vi "AlliGator Extrapolate Multiple Plots.vi"(8 "error in (no error)":errorcluster, 10 "Selected Plots":i32[](array[numeric]), 11 "Selected Plot Info":T1) -> (0 "error out":errorcluster, 1 "Extrapolated Decay Message":string, 3 "Last Extrapolated Decay":cluster{"t Array":dbl[], "IRF Array":dbl[]}, 4 "Single Plot?":bool)   [LabVIEW 2021, in "AlliGator Decay Processing.lvlib"]
doc: "Extrapolated the selected plots."
uses:
  AlliGator Decay Processing.lvlib
  Graphs/XY Graph/XY Graph Selected Plot Info.ctl
  Graphs/XY Graph/XY Graph Refnum.ctl
  <vilib>/Utility/miscctls.llb/LVPoint32TypeDef.ctl
  Strings/Strings.lvlib
  Decay Preprocessing/AlliGator Decay Preprocessing.lvlib
  Graphs/XY Graph/XY Graph Add-Ons.lvlib
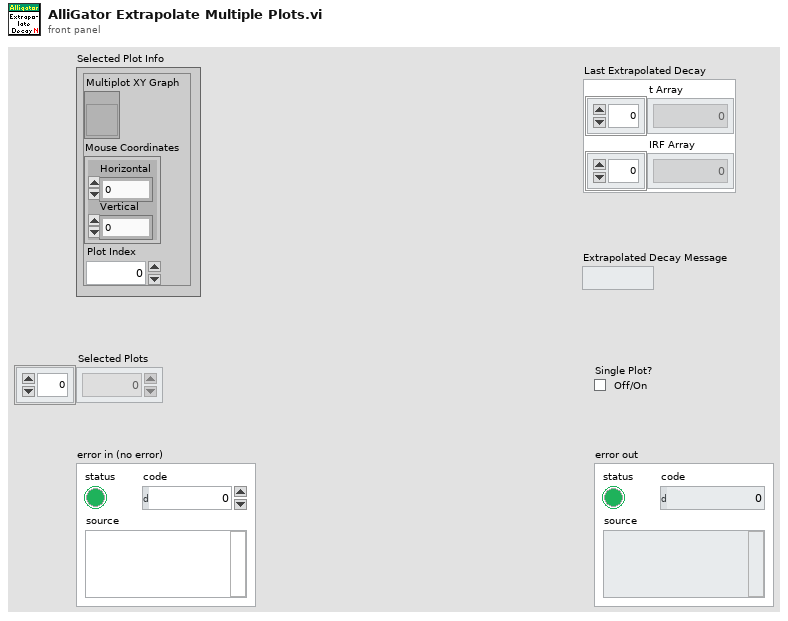
[diagram p1: front panel]
types:
  T1 = typedef "XY Graph Add-Ons.lvlib/XY Graph Selected Plot Info.ctl" = cluster{"Multiplot XY Graph":T2, "Mouse Coordinates":T3, "Plot Index":i32}
  T2 = typedef "XY Graph Add-Ons.lvlib/XY Graph Refnum.ctl" = refnum<vi>
  T3 = typedef "LVPoint32TypeDef.ctl" = cluster{"Horizontal":i32, "Vertical":i32}
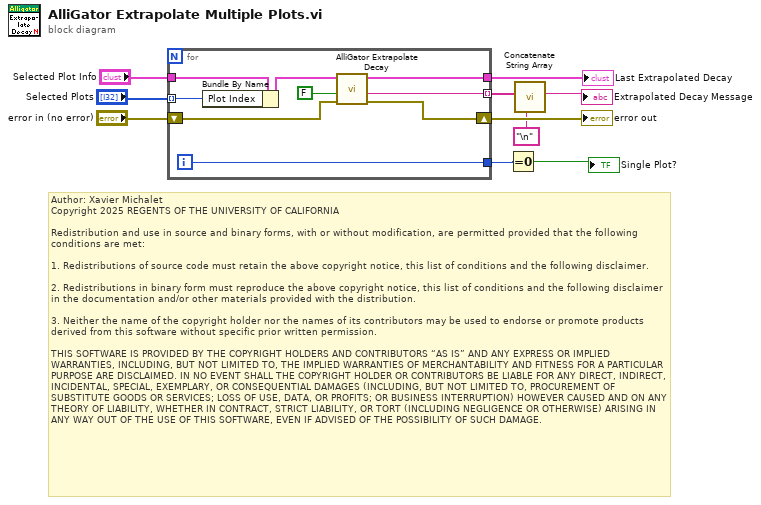
[diagram p0: block diagram]
diagram:
  # "Author: Xavier Michalet\nCopyright 2025 REGENTS OF THE UNIVERSITY OF CALIFORNIA\n\nRedistribution and use in source and binary forms, with or without modification, are permitted provided that the following conditions are met:\n\n1. Redistributions of source code must retain the above copyright notice, this list of conditions and the following disclaimer.\n\n2. Redistributions in binary form must reproduce the above copyright notice, this list of conditions and the following disclaimer in the documentation and/or other materials provided with the distribution.\n\n3. Neither the name of the copyright holder nor the names of its contributors may be used to endorse or promote products derived from this software without specific prior written permission.\n\nTHIS SOFTWARE IS PROVIDED BY THE COPYRIGHT HOLDERS AND CONTRIBUTORS “AS IS” AND ANY EXPRESS OR IMPLIED WARRANTIES, INCLUDING, BUT NOT LIMITED TO, THE IMPLIED WARRANTIES OF MERCHANTABILITY AND FITNESS FOR A PARTICULAR PURPOSE ARE DISCLAIMED. IN NO EVENT SHALL THE COPYRIGHT HOLDER OR CONTRIBUTORS BE LIABLE FOR ANY DIRECT, INDIRECT, INCIDENTAL, SPECIAL, EXEMPLARY, OR CONSEQUENTIAL DAMAGES (INCLUDING, BUT NOT LIMITED TO, PROCUREMENT OF SUBSTITUTE GOODS OR SERVICES; LOSS OF USE, DATA, OR PROFITS; OR BUSINESS INTERRUPTION) HOWEVER CAUSED AND ON ANY THEORY OF LIABILITY, WHETHER IN CONTRACT, STRICT LIABILITY, OR TORT (INCLUDING NEGLIGENCE OR OTHERWISE) ARISING IN ANY WAY OUT OF THE USE OF THIS SOFTWARE, EVEN IF ADVISED OF THE POSSIBILITY OF SUCH DAMAGE."
  n1 = for {
    tunnel: "Selected Plot Info" -> [w19]
    tunnel: [w17] -> w5 mode=indexing
    tunnel: [w15] -> w7
    shift-right: [w16] -> w8
    shift-left: "error in (no error)" -> [w18]
    tunnel: "Selected Plots" -> [w13] mode=indexing
    tunnel: [w12] -> w2
    i -> [w12]
    n2 = Bundle By Name(cluster=w19, "Plot Index"=w13) -> (w14:T1)
    n3 = call "AlliGator Extrapolate Decay.vi"("error in (no error)"=w18, "Replace Plot (T)?"=FALSE, "Selected Plot Info"=w14) -> ("Error Out"=w16:errorcluster, "Message"=w17:string, "Extrapolated Decay"=w15:cluster{"t Array":dbl[], "IRF Array":dbl[]})  [unwired: 6 in]
  }
  "error out" <- w8
  "Last Extrapolated Decay" <- w7
  n4 = Equal To 0?(x=w2) -> (x = 0?=→"Single Plot?":bool)
  n5 = call "Concatenate String Array.vi"("Separator (TAB)"="\n", "String Array"=w5) -> ("Formatted String"=→"Extrapolated Decay Message":string)  [unwired: 9 in]
